vi "OE2031&OE2041_Data Index.vi"(1 "Parameter Type":u16(ring) items=["X", "Y", "R", "θ", "Frequency", "XD1", "YD1", "RD1", "θD1", "XD2", "YD2", "RD2", "θD2", "XD3", "YD3", "RD3", "θD3", "X_Noise", "Y_Noise", "AUXADC1", "AUXADC2", "AUXADC3", "AUXADC4"], 2 "Input Date Array":dbl[](array[numeric])) -> (0 "Parameter":dbl)   [LabVIEW 2011]
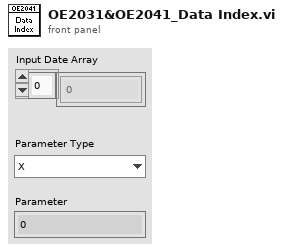
[diagram p1: front panel]
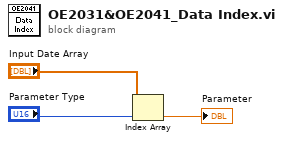
[diagram p0: block diagram]
diagram:
  n1 = Index Array(array="Input Date Array", index="Parameter Type") -> (element=→"Parameter":dbl)
